vi "Handle Command.vi"(8 "error in (no error)":errorcluster, 10 "CMD in":refnum<class "Change Laser Frequency CMD.lvclass">, 11 "Object In":refnum<class>) -> (0 "error out":errorcluster, 1 "Command Successful?":bool, 2 "CMD out":refnum<class "Change Laser Frequency CMD.lvclass">, 3 "Object Out":refnum<class>)   [LabVIEW 2016, in "gPAS Library.lvlib" / "Change Laser Frequency CMD.lvclass"]
doc: "This VI will contain the code used to actually execute the request. If the request is successful, this will be indicated by the boolean output <b>Command Successful?</b>. The boolean output can then be used by the <b>Command Reply</b> which sends a reply if the reply queue is valid."
uses:
  Change Laser Frequency CMD.lvclass
  nPAS.lvclass
  C:/Program Files (x86)/National Instruments/LabVIEW 2016/vi.lib/MSR Consulting, LLC/General Reuse/Instrument/Instrument.lvclass
  C:/Program Files (x86)/National Instruments/LabVIEW 2016/vi.lib/MSR Consulting, LLC/General Reuse/PAS/Main/PAS.lvclass
  <vilib>/MSR Consulting, LLC/General Reuse/Instrument/Instrument.lvclass/Instrument.ctl
  nPAS.lvclass/nPAS.ctl
  Change Laser Frequency CMD.lvclass/Change Laser Frequency CMD.ctl
  <vilib>/MSR Consulting, LLC/General Reuse/PAS/Cell/PAS Cell.lvclass/PAS Cell.ctl
  <vilib>/MSR Consulting, LLC/General Reuse/PAS/Cell/Write Mod Freq.vi
  <vilib>/MSR Consulting, LLC/General Reuse/Instrument/Read Log Session.vi
  Accessors/Read hFPGA.vi
  <vilib>/MSR Consulting, LLC/General Reuse/Instrument/Read ExtCom.vi
  <vilib>/MSR Consulting, LLC/General Reuse/PAS/Main/Read Cells.vi
  <vilib>/Utility/error.llb/Error Cluster From Error Code.vi
  <vilib>/rvi/errors/niLvFpgaAdjustHostInterfaceError.vi
  <vilib>/MSR Consulting, LLC/General Reuse/PAS/Main/Write Cells.vi
  <vilib>/MSR Consulting, LLC/General Reuse/Session APIs/_Session Fwk/Session - Root.lvclass
  <vilib>/MSR Consulting, LLC/General Reuse/PAS/Cell/PAS Cell.lvclass
  <vilib>/rvi/interface/nirviReadWriteControl/nirviReadWriteControl.xnode
  FPGA Ref.ctl
  FPGA Bitfiles/NickIO.lvbitx
  <vilib>/MSR Consulting, LLC/General Reuse/Session APIs/Session Log/System Log.lvclass
  NiFpgaLv.dll
  Session/Raw FPGA/FPGA Session.lvclass
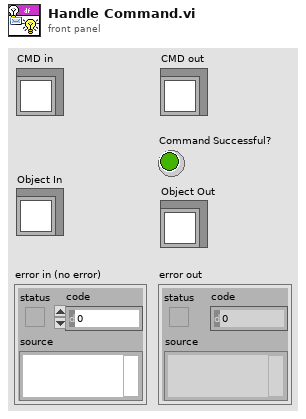
[diagram p1: front panel]
types:
  T1 = typedef "Session - Root.lvclass/Session Handle.ctl" = refnum<data-value>
  T2 = typedef "FPGA Ref.ctl" = refnum<k20>
  T3 = cluster{"tag":string, "section":string, "data":variant}
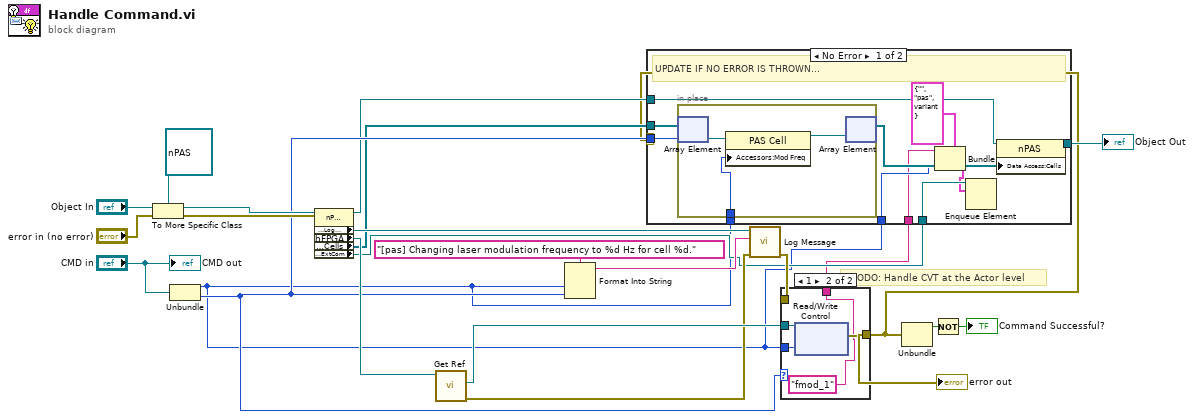
[diagram p0: block diagram]
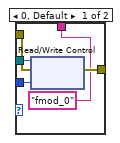
[diagram p3: hidden frame]
diagram:
  # "#TODO: Handle CVT at the Actor level"
  n1 = To More Specific Class(target class=refnum<class "nPAS.lvclass"> refnum ("nPAS"), reference="Object In", error in="error in (no error)") -> (specific class reference=w20:refnum<class "nPAS.lvclass">, error out=w19:errorcluster)
  n2 = Unbundle("CMD in") -> (w1:u32, w8:u8)
  n3 = property class="nPAS"(reference=w20, error in=w19) -> (reference out=w6:refnum<class "nPAS.lvclass">, "Accessors:Log Session"=w18:T1, "hFPGA"=w11:T1, "Data Access:Cells"=w7:refnum<class "PAS Cell.lvclass">[], "Accessors:ExtCom"=w3:refnum<queue>)  [unwired: 1 out]
  n4 = call "Get Ref.vi"("Hanlde Out"=w11) -> ("error out"=w9:errorcluster, "FPGA Ref"=w10:T2)  [unwired: 8 in, 1 out]
  n5 = Format Into String(format string="[pas] Changing laser modulation frequency to %d Hz for cell %d.", w1, w8) -> (resulting string=w16:string)  [unwired: 2 in, 1 out]
  n6 = call <vilib>:"Log Message.vi"("error in"=w9, "MSG In"=w16, "session in"=w18) -> ("error out"=w15:errorcluster)  [unwired: 7 in, 1 out]
  n7 = case shown="1" w8 {
    tunnel: w1 -> [w28 w31]
    tunnel: w15 -> [w27 _]
    tunnel: [w26 w30] -> w4
    tunnel: w10 -> [w25 w32]
    tunnel: ["fmod_0" ("tag") "fmod_1" ("tag")] -> w2
    frame 0, Default {
      n8 = xnode "Read/Write Control"("FPGA VI Reference In"=w25, "error in"=w27, "f0"=w28) -> ("error out"=w26:errorcluster)  [unwired: 1 out]
    }
    frame 1 {
      n9 = xnode "Read/Write Control"("FPGA VI Reference In"=w32, "f1"=w31) -> ("error out"=w30:errorcluster)  [unwired: 1 in, 1 out]
    }
  }
  "error out" <- w4
  n10 = case shown="No Error" w4 {
    tunnel: w8 -> [w43 _]
    tunnel: w7 -> [w42 _]
    tunnel: w1 -> [w41 _]
    tunnel: w6 -> [w40 w47]
    tunnel: [w39 w47] -> w5
    tunnel: w3 -> [w37 _]
    tunnel: w2 -> [w33 _]
    tunnel: w1 -> [w35 _]
    frame No Error {
      # "UPDATE IF NO ERROR IS THROWN..."
      n11 = in-place {
        in-place-border: w41 -> [w45]
        n12 = in-place-array #1(w42, w43) -> (w46:refnum<class "PAS Cell.lvclass">)
        n13 = property class="PAS Cell"(reference=w46, "Accessors:Mod Freq"=w45) -> (reference out=w44:refnum<class "PAS Cell.lvclass">)  [unwired: 1 in, 1 out]
        n14 = in-place-array #1(w44) -> (w38:refnum<class "PAS Cell.lvclass">[])  [unwired: 1 out]
      }
      n15 = Bundle(cluster=T3 {"tag"="", "section"="pas", "data"=variant} ("element"), "tag"=w33, "data"=w35) -> (w34:T3)  [unwired: 1 in]
      n16 = Enqueue Element(queue=w37, element=w34) -> ()  [unwired: 2 in, 3 out]
      n17 = property class="nPAS"(reference=w40, "Data Access:Cells"=w38) -> (reference out=w39:refnum<class "nPAS.lvclass">)  [unwired: 1 in, 1 out]
    }
    frame Error {
    }
  }
  "Object Out" <- w5
  n18 = Unbundle(w4) -> ("status"=w13:bool)  [unwired: 2 out]
  n19 = Not(x=w13) -> (.not. x?=→"Command Successful?":bool)
  "CMD out" <- "CMD in"
